vi "Discrete Control systemn with OPC UA.vi"() -> ()   [LabVIEW 2025]
uses:
  <vilib>/OPCUA/controls/NodeId.ctl
  <vilib>/OPCUA/controls/Write Status.ctl
  <vilib>/OPCUA/client/Connect2.vi
  <vilib>/OPCUA/client/Multiple Write Double.vi
  <vilib>/OPCUA/NI OPC UA Client.lvlib
panel:
  in  "Server Endpoint URL":string="opc.tcp://LAPTOP-S9B2BQJO:49580"
  out "U [v]":dbl
  in  "SetPoint [C]":dbl
  in  "PI parameters":cluster{"Kp [V/C]":dbl, "Ti [s]":dbl}={"Kp [V/C]"=0.5, "Ti [s]"=4.0}
  out "Waveform Chart":dbl(graph)
  out "Process value[C]":dbl format="%#_3g"
  in  "Model parameters":cluster{"K":dbl, "T":dbl}={"K"=8.0, "T"=4.0}
  in  "Ts [s]":dbl=0.1
  in  "Stop":bool
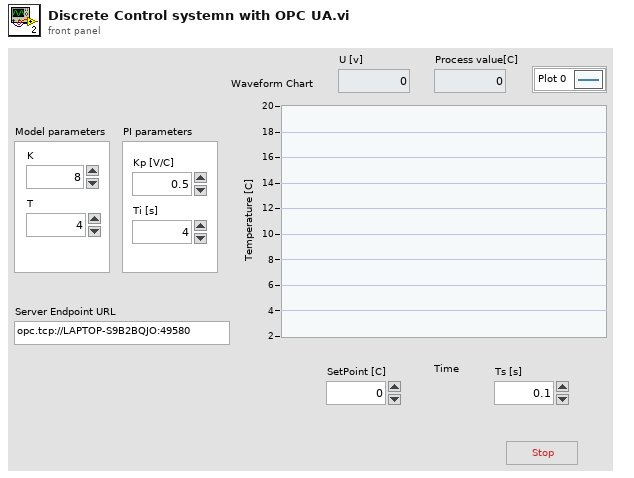
[diagram p1: front panel]
types:
  T1 = cluster{"message mode":enum16{"None", "Sign", "Sign and Encrypt"}, "security":enum16{"Basic256Sha256", "Aes128Sha256RsaOaep", "Aes256Sha256RsaPss"}}
  T2 = typedef "OPC UA Client Refnum.ctl" = refnum<k21>
  T3 = typedef "NodeId.ctl" = string
  T4 = typedef "Write Status.ctl" = u32
  T5 = cluster{"node ID":T3, "value":dbl, "timestamp (current time)":timestamp, "node status":T4}
  T6 = cluster{"node ID":T3, "value":dbl, "timestamp (current time)":timestamp, "node status":T4}[]
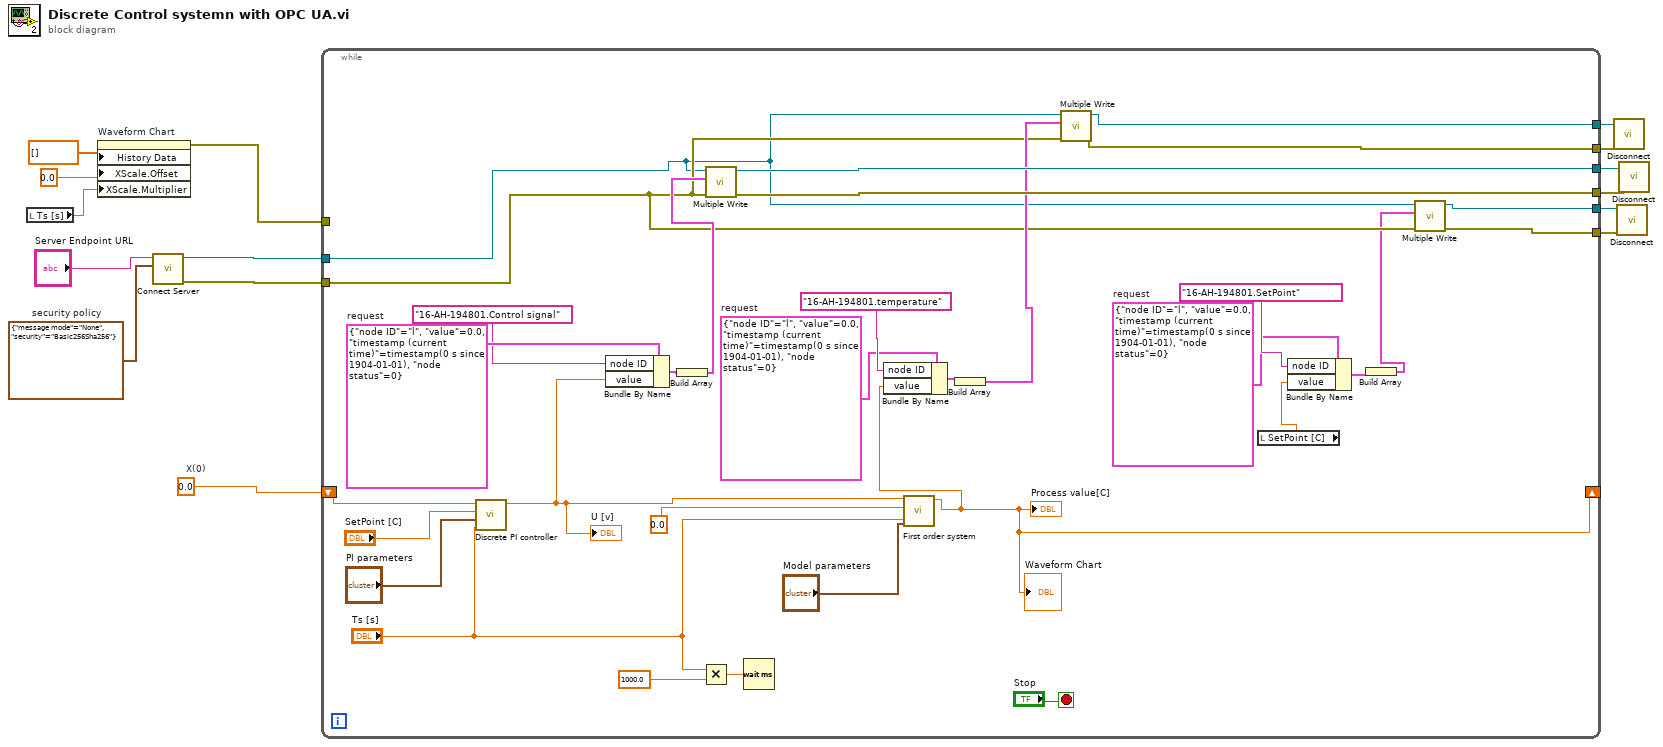
[diagram p0: block diagram]
diagram:
  w9 = T1 {"message mode"=enum."None", "security"=enum."Basic256Sha256"}  # security policy
  w11 = 0.0  # X(0)
  n1 = local read "Ts [s]"() -> (w12:dbl)
  n2 = property on="Waveform Chart" class="WFChart (strict)"("History Data"=dbl[] [], "XScale.Offset"=0.0 ("X Scale.Offset and Multiplier:Offset"), "XScale.Multiplier"=w12) -> (error out=w14:errorcluster)  [unwired: 2 in, 1 out]
  n3 = call-poly <vilib>:"Connect Server.vi"("security policy"=w9, "server endpoint URL"="Server Endpoint URL") -> ("error out"=w8:errorcluster, "OPC UA client refnum out"=w7:T2)  [unwired: 7 in, 1 out]
  n4 = while {
    tunnel: w14 -> [_]
    shift-right: [w29] -> _
    shift-left: w11 -> [w42]
    tunnel: w8 -> [w22]
    tunnel: w7 -> [w21]
    tunnel: [w38] -> w6
    tunnel: [w37] -> w5
    tunnel: [w27] -> w4
    tunnel: [w26] -> w3
    tunnel: [w17] -> w2
    tunnel: [w16] -> w1
    stop <- "Stop" stop-if-true
    w20 = T5 {"node ID"="l", "value"=0.0, "timestamp (current time)"=timestamp(0 s since 1904-01-01), "node status"=0}  # request
    w28 = T5 {"node ID"="l", "value"=0.0, "timestamp (current time)"=timestamp(0 s since 1904-01-01), "node status"=0}  # request
    w36 = T5 {"node ID"="l", "value"=0.0, "timestamp (current time)"=timestamp(0 s since 1904-01-01), "node status"=0}  # request
    n5 = call "Discrete PI controller.vi"("Ts [s]"="Ts [s]", "PI parameters"="PI parameters", "SetPoint [C]"="SetPoint [C]", "Process value [C]"=w42) -> ("U [v]"=w34:dbl)  [unwired: 7 in]
    "U [v]" <- w34
    n6 = Bundle By Name "Bundle By Name"(cluster=w36, "node ID"=T3 "16-AH-194801.Control signal", "value"=w34) -> (w33:T5)
    n7 = Build Array(w33) -> (w32:T6)
    n8 = Multiply(x="Ts [s]", y=1000.0) -> (x*y=w45:dbl)
    n9 = call-poly <vilib>:"Multiple Write.vi"("error in (no error)"=w22, "requests"=w32, "OPC UA client refnum in"=w21) -> ("error out"=w37:errorcluster, "OPC UA client refnum out"=w38:T2)  [unwired: 5 in, 2 out]
    n10 = Wait (ms)(milliseconds to wait=w45) -> ()  [unwired: 1 out]
    n11 = call "First order system.vi"("Model parameters"="Model parameters", "Ts"="Ts [s]", "x(0)"=0.0, "u"=w34) -> ("X"=w29:dbl)  [unwired: 7 in]
    "Process value[C]" <- w29
    "Waveform Chart" <- w29
    n12 = Bundle By Name "Bundle By Name"(cluster=w28, "node ID"=T3 "16-AH-194801.temperature", "value"=w29) -> (w31:T5)
    n13 = Build Array(w31) -> (w25:T6)
    n14 = call-poly <vilib>:"Multiple Write.vi"("error in (no error)"=w22, "requests"=w25, "OPC UA client refnum in"=w21) -> ("error out"=w27:errorcluster, "OPC UA client refnum out"=w26:T2)  [unwired: 5 in, 2 out]
    n15 = local read "SetPoint [C]"() -> (w23:dbl)
    n16 = Bundle By Name "Bundle By Name"(cluster=w20, "node ID"=T3 "16-AH-194801.SetPoint", "value"=w23) -> (w19:T5)
    n17 = Build Array(w19) -> (w18:T6)
    n18 = call-poly <vilib>:"Multiple Write.vi"("error in (no error)"=w22, "requests"=w18, "OPC UA client refnum in"=w21) -> ("error out"=w16:errorcluster, "OPC UA client refnum out"=w17:T2)  [unwired: 5 in, 2 out]
  }
  n19 = call <vilib>:"Disconnect.vi"("error in (no error)"=w4, "OPC UA client refnum in"=w3) -> ()  [unwired: 9 in, 1 out]
  n20 = call <vilib>:"Disconnect.vi"("error in (no error)"=w1, "OPC UA client refnum in"=w2) -> ()  [unwired: 9 in, 1 out]
  n21 = call <vilib>:"Disconnect.vi"("error in (no error)"=w5, "OPC UA client refnum in"=w6) -> ()  [unwired: 9 in, 1 out]
